vi "PCO_DoWhiteBalance.vi"(8 "error in (no error)":errorcluster {"code" format="%x"}, 10 "wMode":u16(ring)=1 items=["start white balance process"=1], 11 "ph":u64) -> (0 "error out":errorcluster {"code" format="%x"}, 2 "ErrorMessage":i32 format="%x", 3 "ph out":u64)   [LabVIEW 2019, in "SDK.lvlib" / "SpecialCommandsDimax_HDSDI.lvlib"]
doc: "<b>Description:</b>\nThis function does start a white balance calculation process. The function must only be called, when images are transmitted to the HD-SDI interface and one of the color formats is selected. The function does return immediately. The camera uses a 50% image region in the center of the image to calculate new values for wColorTemp and sTint of the PCO_Image_ColorSet structure.\n\n<b>Supported camera type:</b>\npco.dimax with HD-SDI interface\n\n<b>Descriptor dependency:</b>\nNone"
uses:
  SpecialCommandsDimax_HDSDI.lvlib
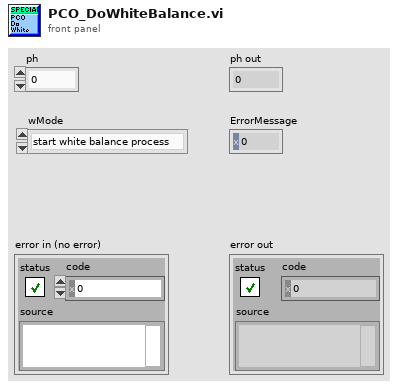
[diagram p1: front panel]
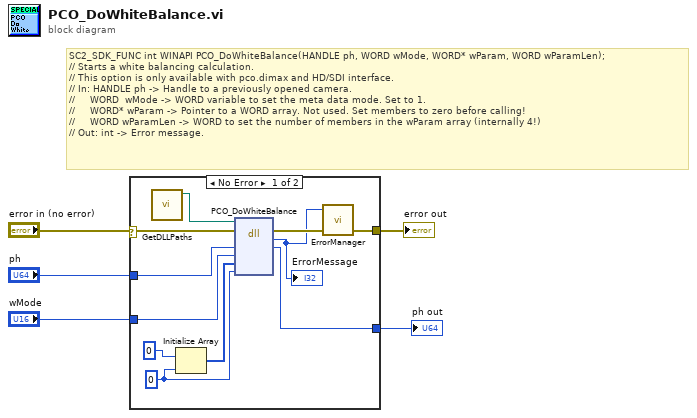
[diagram p0: block diagram]
diagram:
  # "SC2_SDK_FUNC int WINAPI PCO_DoWhiteBalance(HANDLE ph, WORD wMode, WORD* wParam, WORD wParamLen);\n// Starts a white balancing calculation.\n// This option is only available with pco.dimax and HD/SDI interface.\n// In: HANDLE ph -> Handle to a previously opened camera.\n//     WORD  wMode -> WORD variable to set the meta data mode. Set to 1.\n//     WORD* wParam -> Pointer to a WORD array. Not used. Set members to zero before calling!\n//     WORD wParamLen -> WORD to set the number of members in the wParam array (internally 4!)\n// Out: int -> Error message."
  n1 = case shown="No Error" "error in (no error)" {
    selector: "error in (no error)" -> [w10 w18]
    tunnel: "ph" -> [w16 w17]
    tunnel: [w15 w17] -> w4
    tunnel: "wMode" -> [w14 _]
    tunnel: [w9 w18] -> w2
    frame No Error {
      w12 = u16 0 ("wParamLen")
      n2 = call "GetDLLPaths.vi"() -> ("SC2_Cam_Path"=w6:path)  [unwired: 8 in, 3 out]
      n3 = Initialize Array(u16 0, w12) -> (w11:u16[])
      n4 = dll-call lib="?" fn="PCO_DoWhiteBalance"(path in=w6, error in=w10, "ph"=w16, "wMode"=w14, "wParam"=w11, "wParamLen"=w12) -> (error out=w8:errorcluster, "return type"=w7:i32, "ph"=w15:u64)  [unwired: 4 in, 1 out]
      "ErrorMessage" <- w7
      n5 = call "ErrorManager.vi"("error in (no error)"=w8, "error code"=w7) -> ("error out"=w9:errorcluster)  [unwired: 2 in, 1 out]
    }
    frame Error {
    }
  }
  "ph out" <- w4
  "error out" <- w2
